vi "Send User Dialog Message.vi"(8 "Error In":errorcluster, 11 "Error String":string) -> (0 "Error Out":errorcluster)   [LabVIEW 2015]
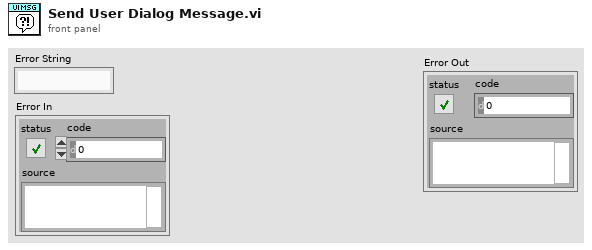
[diagram p1: front panel]
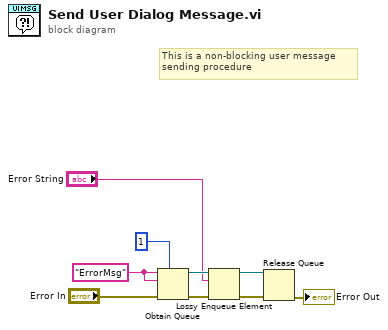
[diagram p0: block diagram]
diagram:
  w8 = "ErrorMsg" ("name (unnamed)")
  # "This is a non-blocking user message \nsending procedure"
  n1 = Obtain Queue(max queue size (-1, unlimited)=1, name (unnamed)=w8, element data type=w8, error in (no error)="Error In") -> (queue out=w7:refnum<queue>, error out=w6:errorcluster)  [unwired: 1 in, 1 out]
  n2 = Lossy Enqueue Element(queue=w7, element="Error String", error in (no error)=w6) -> (queue out=w3:refnum<queue>, error out=w4:errorcluster)  [unwired: 2 out]
  n3 = Release Queue(queue=w3, error in (no error)=w4) -> (error out=→"Error Out":errorcluster)  [unwired: 1 in, 2 out]
